vi "WFAppend.vi"   [LabVIEW 2013]
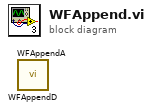
[diagram p0: block diagram]
diagram:
  n1 = call "WFAppendD.vi"() -> ()  [unwired: 18 in, 2 out]
  n2 = call "WFAppendA.vi"() -> ()  [unwired: 18 in, 2 out]
